vi "Q3_saving.vi"() -> ()   [LabVIEW 2020]
uses:
  54402a8a-6335-4590-be97-694ebf0c10c0.vi
  <vilib>/Array/Sort 2D Array - Pop Stack.vi
  <vilib>/Array/Sort 2D Array - Push Stack.vi
  54402a8a-6335-4590-be97-694ebf0c10c0.vi/269d4b3b-47f5-49e3-8884-44851e4dd9d5.vi
  54402a8a-6335-4590-be97-694ebf0c10c0.vi/6d99389c-673d-4efb-bf33-19b32bcf4cf8.vi
  <vilib>/Utility/file.llb/Read Delimited Spreadsheet (DBL).vi
  <vilib>/Utility/file.llb/Write Delimited Spreadsheet (DBL).vi
panel:
  in  "file path for saving 3b":path
  out "subarray 2":dbl[](array[numeric])
  out "subarray":dbl[](array[numeric])
  out "Slope":dbl
  out "Intercept":dbl
  out "3c":cluster{dbl[], dbl[]}[](graph)
  out "3b":dbl[][](array[numeric])
  out "3a":dbl[][](array[numeric])
  out "3a":cluster{"Y":dbl[], "Y":dbl[]}[](graph)
  in  "file path (dialog if empty)":path
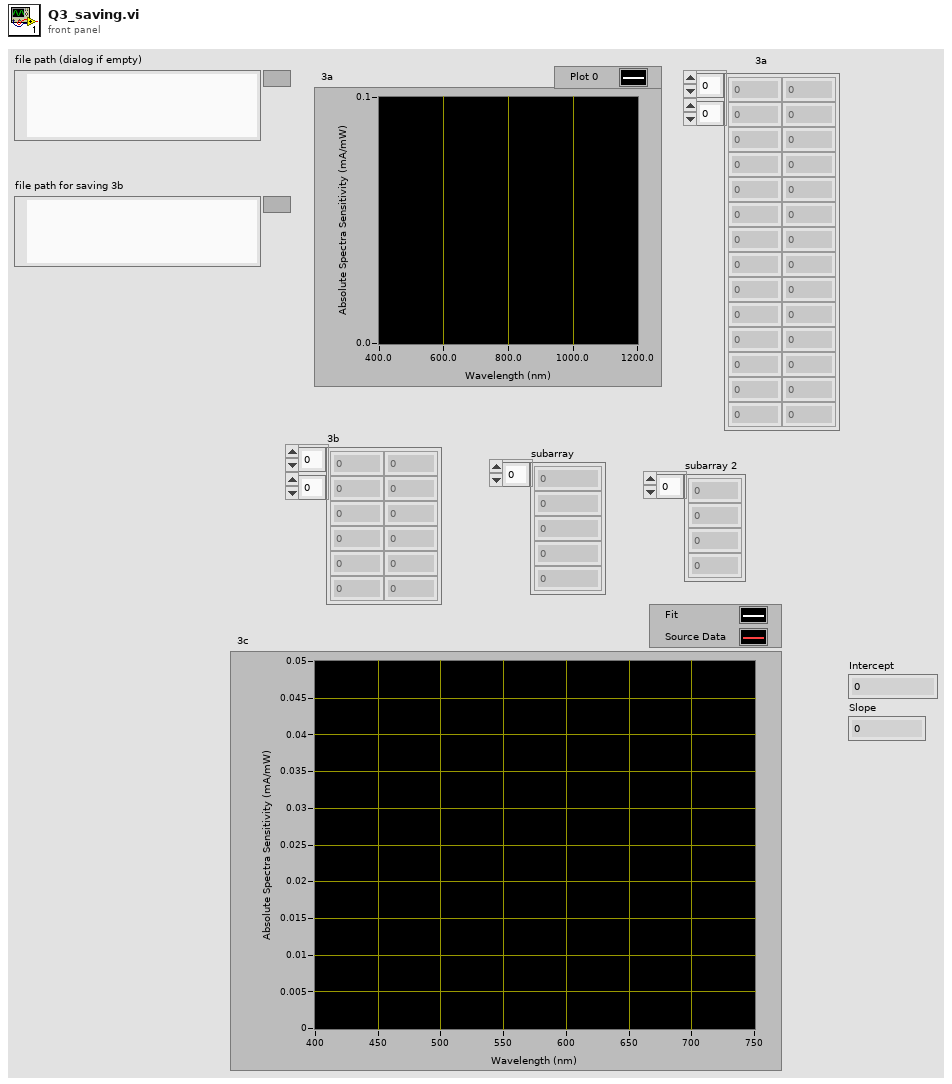
[diagram p1: front panel]
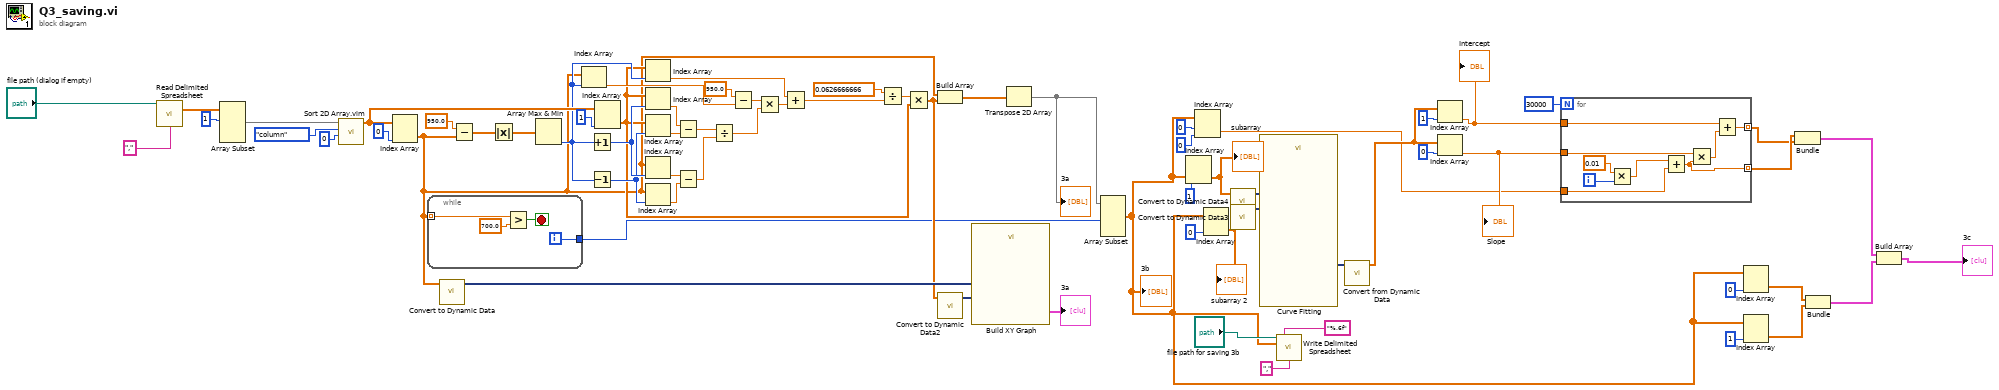
[diagram p0: block diagram]
diagram:
  n1 = call-poly <vilib>:"Read Delimited Spreadsheet.vi"("file path (dialog if empty)"="file path (dialog if empty)", "delimiter (\\t)"="," ("delimiter (\\t)")) -> ("all rows"=w66:dbl[][])  [unwired: 8 in, 5 out]
  n2 = Array Subset(array=w66, index (row)=1 ("index")) -> (w33:dbl[][])  [unwired: 3 in]
  n3 = call "Sort 2D Array.vim"("index"=0, "dimension to index (column)"=enum16{"column", "row"}."column", "2D array"=w33) -> ("sorted 2D array"=w61:dbl[][])  [unwired: 7 in, 1 out]
  n4 = Index Array(array=w61, index (col)=0 ("disabled index (col)")) -> (element=w32:dbl[])  [unwired: 1 in]
  n5 = while {
    tunnel: w32 -> [w71] mode=indexing
    tunnel: [w70] -> w30
    i -> [w70]
    stop <- w72 stop-if-true
    n6 = Greater?(x=w71, y=700.0) -> (0:w72:bool)
  }
  n7 = call "Convert to Dynamic Data"("Array"=w32) -> ("Dynamic Data Type"=w62:dynamicdata)  [unwired: 3 in]
  n8 = Subtract(x=950.0 ("y"), y=w32) -> (x-y=w57:dbl[])
  n9 = Absolute Value(x=w57) -> (abs(x)=w56:dbl[])
  n10 = Array Max & Min(array=w56) -> (min index (indices)=w48:i32)  [unwired: 3 out]
  n11 = Index Array(array=w32, index=w48) -> (element=w43:dbl)
  n12 = Increment(x=w48) -> (x+1=w55:i32)
  n13 = Decrement(x=w48) -> (x-1=w54:i32)
  n14 = Index Array(array=w61, index (col)=1 ("disabled index (col)")) -> (element=w39:dbl[])  [unwired: 1 in]
  n15 = Index Array(array=w39, index=w48) -> (element=w49:dbl)
  n16 = Index Array(array=w39, index=w55) -> (element=w51:dbl)
  n17 = Index Array(array=w39, index=w54) -> (element=w50:dbl)
  n18 = Index Array(array=w32, index=w55) -> (element=w53:dbl)
  n19 = Index Array(array=w32, index=w54) -> (element=w52:dbl)
  n20 = Subtract(x=w51, y=w50) -> (x-y=w36:dbl)
  n21 = Subtract(x=w53, y=w52) -> (x-y=w37:dbl)
  n22 = Divide(x=w36, y=w37) -> (x/y=w46:dbl)
  n23 = Subtract(x=950.0 ("y"), y=w43) -> (x-y=w47:dbl)
  n24 = Multiply(x=w47, y=w46) -> (x*y=w45:dbl)
  n25 = Add(x=w49, y=w45) -> (x+y=w42:dbl)
  n26 = Divide(x=0.0626666666, y=w42) -> (x/y=w40:dbl)
  n27 = Multiply(x=w40, y=w39) -> (x*y=w35:dbl[])
  n28 = Build Array(w32, w35) -> (w34:dbl[][])
  n29 = call "Convert to Dynamic Data2"("Array"=w35) -> ("Dynamic Data Type"=w38:dynamicdata)  [unwired: 3 in]
  n30 = call "Build XY Graph"("Y Input"=w38, "X Input"=w62) -> ("XY Graph"=→"3a":cluster{"X":dbl[], "Y":dbl[]}[])  [unwired: 8 in, 1 out]
  n31 = Transpose 2D Array(2D array=w34) -> (transposed array=w31:dbl[][])
  "3a" <- w31
  n32 = Array Subset(array=w31, length (row)=w30) -> (w3:dbl[][])  [unwired: 3 in]
  "3b" <- w3
  n33 = Index Array(array=w3, index (col)=1 ("disabled index (col)")) -> (element=w11:dbl[])  [unwired: 1 in]
  "subarray" <- w11
  n34 = Index Array(array=w3, index (row)=0, index (col)=0 ("disabled index (col)")) -> (element=w7:dbl)
  n35 = Index Array(array=w3, index (col)=0 ("disabled index (col)")) -> (element=w13:dbl[])  [unwired: 1 in]
  "subarray 2" <- w13
  n36 = call "Convert to Dynamic Data4"("Array"=w11) -> ("Dynamic Data Type"=w10:dynamicdata)  [unwired: 3 in]
  n37 = call "Convert to Dynamic Data3"("Array"=w13) -> ("Dynamic Data Type"=w12:dynamicdata)  [unwired: 3 in]
  n38 = call "Curve Fitting"("Locations"=w12, "Signals"=w10) -> ("general LS coefficients"=w29:dynamicdata)  [unwired: 5 in, 4 out]
  n39 = call-poly <vilib>:"Write Delimited Spreadsheet.vi"("file path (dialog if empty)"="file path for saving 3b", "format (%.3f)"="%.6f", "2D data"=w3, "delimiter (\\t)"="," ("delimiter (\\t)")) -> ()  [unwired: 10 in, 2 out]
  n40 = call "Convert from Dynamic Data"("Dynamic Data Type"=w29) -> ("Array"=w28:dbl[])  [unwired: 3 in]
  n41 = Index Array(array=w28, index=1) -> (element=w6:dbl)
  "Intercept" <- w6
  n42 = Index Array(array=w28, index=0) -> (element=w23:dbl)
  "Slope" <- w23
  n43 = for {
    N: 30000 -> [_]
    tunnel: w23 -> [w82]
    tunnel: [w78] -> w21 mode=indexing
    tunnel: [w76] -> w22 mode=indexing
    tunnel: w7 -> [w75]
    tunnel: w6 -> [w74]
    i -> [w81]
    n44 = Multiply(x=0.01, y=w81) -> (x*y=w77:dbl)
    n45 = Add(x=w77, y=w75) -> (x+y=w76:dbl)
    n46 = Multiply(x=w82, y=w76) -> (x*y=w79:dbl)
    n47 = Add(x=w74, y=w79) -> (x+y=w78:dbl)
  }
  n48 = Index Array(array=w3, index (col)=0 ("disabled index (col)")) -> (element=w18:dbl[])  [unwired: 1 in]
  n49 = Index Array(array=w3, index (col)=1 ("disabled index (col)")) -> (element=w17:dbl[])  [unwired: 1 in]
  n50 = Bundle(w22, w21) -> (w15:cluster{dbl[], dbl[]})  [unwired: 1 in]
  n51 = Bundle(w18, w17) -> (w16:cluster{dbl[], dbl[]})  [unwired: 1 in]
  n52 = Build Array(w15, w16) -> (→"3c":cluster{dbl[], dbl[]}[])
